vi "AlGaInPAs_prep_v00.vi"(2 "Debug Mode":bool, 3 "Elapsed Time(s)":dbl, 4 "State":enum16{"Edit", "Start", "Run", "End", "Idle"}(ring), 5 "Argument List In":string[](array[string])) -> (0 "Status Out":string, 1 "Argument List Out":string[](array[string]))   [LabVIEW 2011]
panel:
  out "AsH3?":bool
  out "PH3?":bool
  out "In?":bool
  out "Ga?":bool
  out "Al?":bool
  in  "Prep As":bool caption="Pre-run"
  out "Prep P":bool caption="Pre-run"
  in  "Prep In":bool caption="Pre-run"
  in  "Prep Ga":bool caption="Pre-run"
  in  "run_time":dbl caption="run time (s)"
  in  "prep_time":dbl caption="pre-run time (s)"
  in  "Prep Al":bool caption="Pre-run"
  in  "Run As":bool caption="Run"
  in  "AsH3 Flow":dbl caption="AsH3 Flow (0-10 sccm)" format="%.2f"
  in  "P Flow":dbl caption="P Flow (0-100 sccm)" format="%.2f"
  in  "Run P":bool caption="Run"
  in  "In Flow":dbl caption="In Flow (0-100 sscm)" format="%.2f"
  in  "Run In":bool caption="Run"
  in  "Run Ga":bool caption="Run"
  in  "Ga Flow":dbl caption="Ga Flow (0-10 sscm)" format="%.2f"
  in  "Run Al":bool caption="Run"
  in  "Al Flow":dbl caption="Al Flow (0-100 sscm)" format="%.2f"
  in  "Cancel":bool
  in  "OK":bool
  out "tTotal(s) 2":dbl
  out "tphase(s)":dbl[](array[numeric])
  out "phase":i32
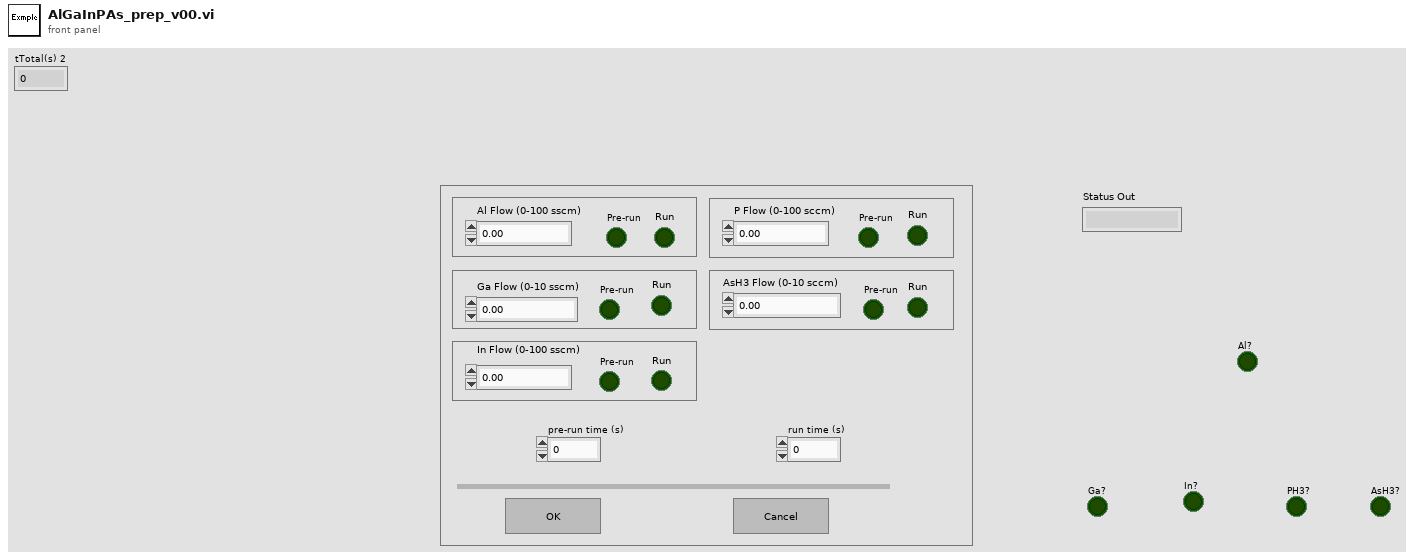
[diagram p1: front panel]
types:
  T1 = enum16{"Discrete", "Continuous", "Instantaneous"}
  T2 = enum32{"Invalid", "Default", "Floating", "Floating/Auto-Hide", "Modal"}
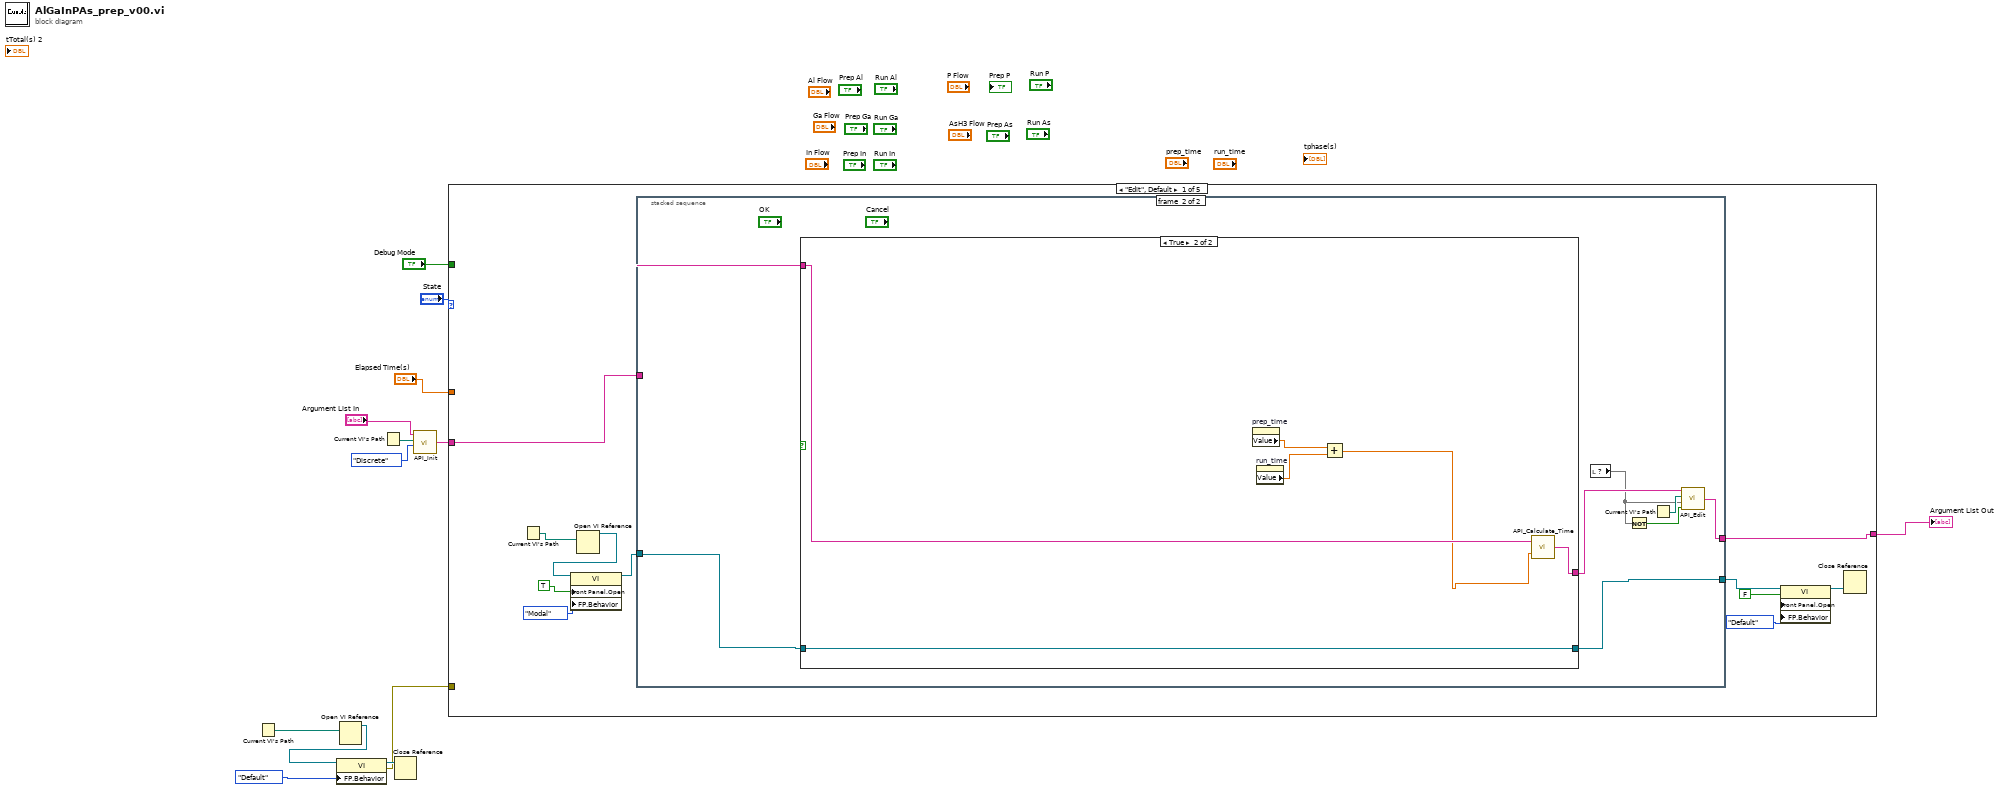
[diagram p0: block diagram]
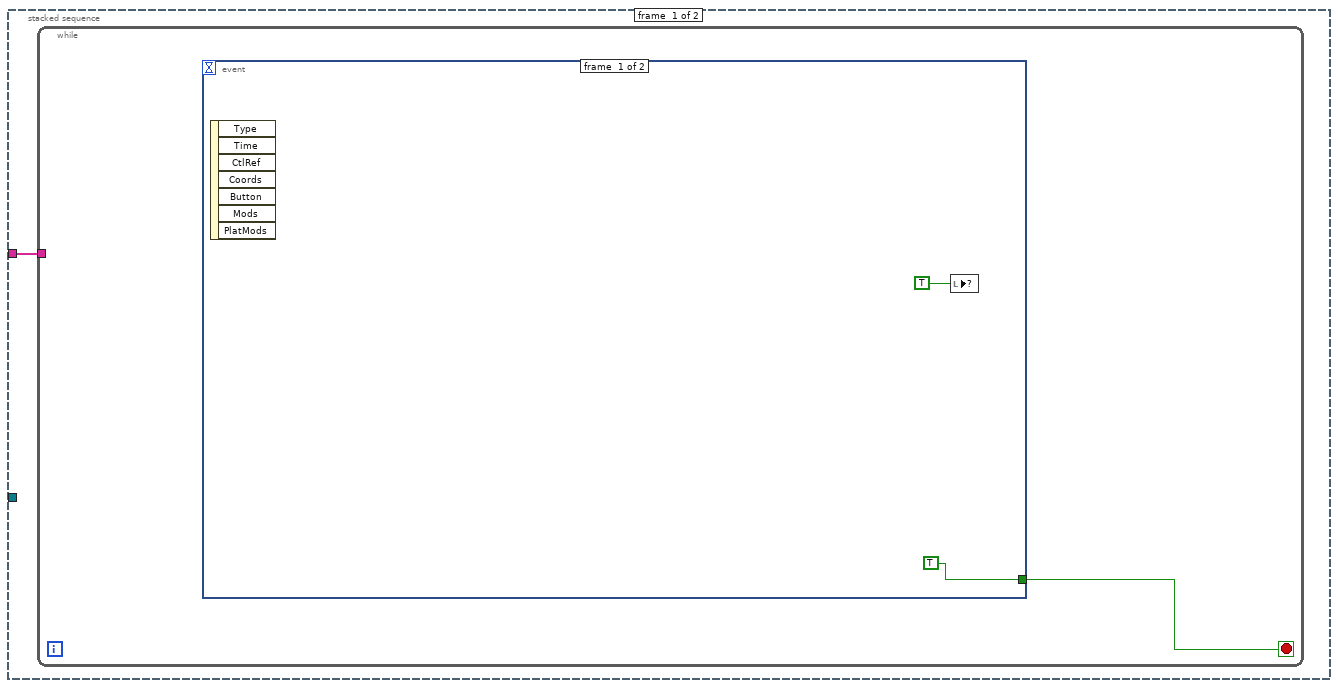
[diagram p2: hidden frame]
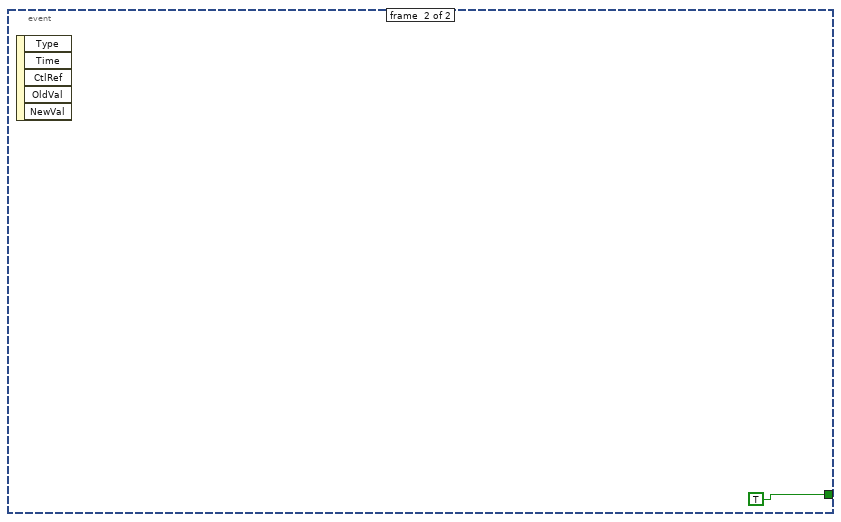
[diagram p3: hidden frame]
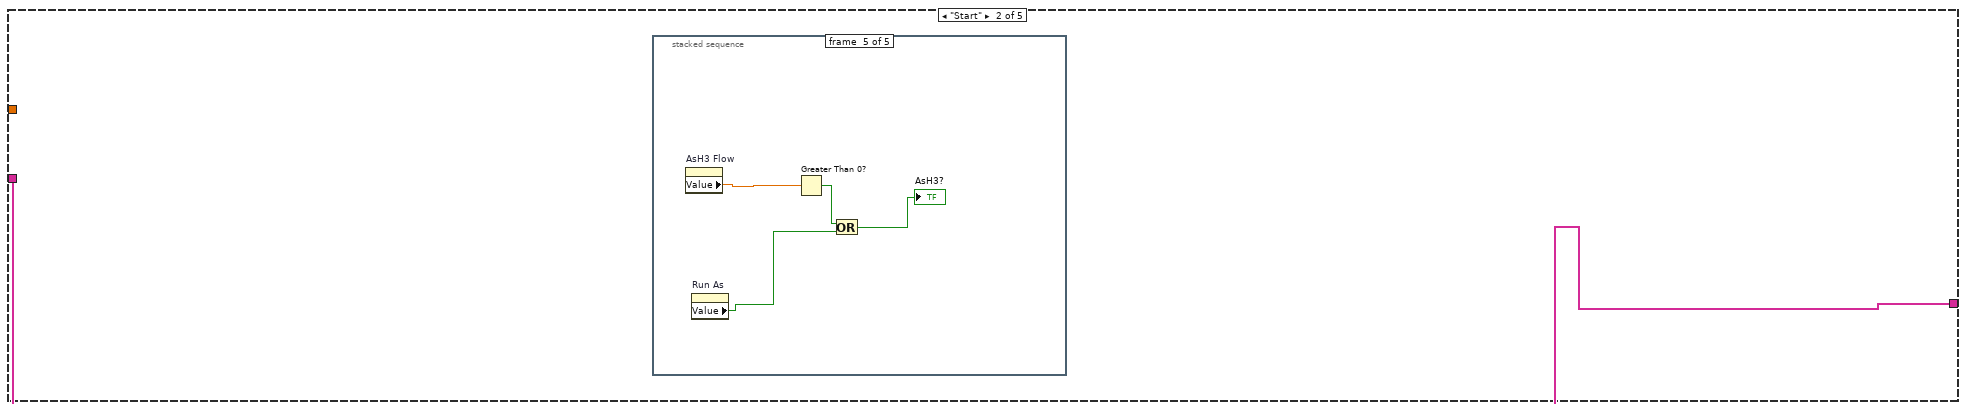
[diagram p5: hidden frame]
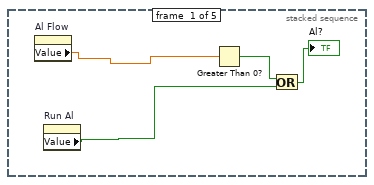
[diagram p6: hidden frame]
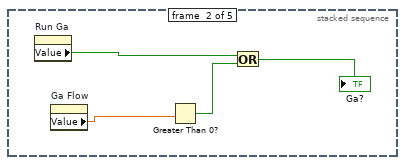
[diagram p7: hidden frame]
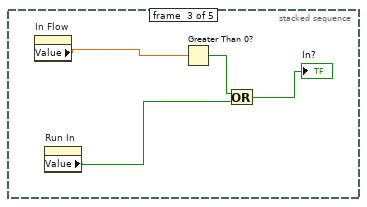
[diagram p8: hidden frame]
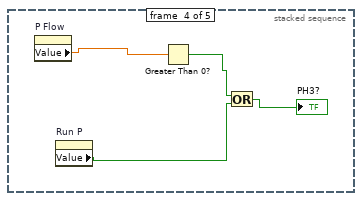
[diagram p9: hidden frame]
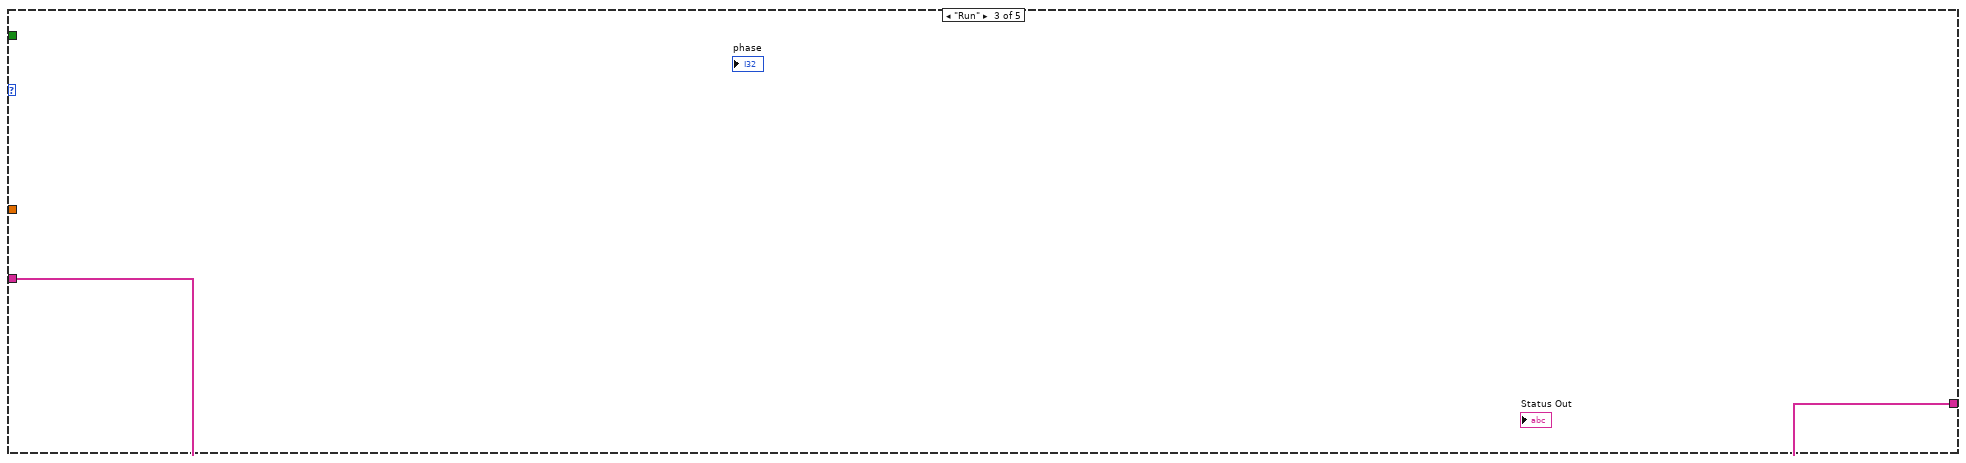
[diagram p10: hidden frame]
diagram:
  n1 = Current VI's Path() -> (path=w9:path)
  n2 = Open VI Reference(vi path=w9) -> (vi reference=w8:refnum<vi>)  [unwired: 1 in, 5 out]
  n3 = property class="VI"(reference=w8, "FP.Behavior"=T2."Default" ("Front Panel Window:Behavior")) -> (reference out=w6:refnum<vi>, error out=w5:errorcluster)  [unwired: 1 in]
  n4 = Current VI's Path() -> (path=w4:path)
  n5 = Close Reference(reference=w6) -> ()  [unwired: 1 in, 1 out]
  n6 = call "API_Init.vi"("API Mode"=T1."Discrete", "VI Path"=w4, "Argument List In"="Argument List In") -> ("Argument List Out"=w1:string[])  [unwired: 1 in]
  n7 = case shown="\"Edit\", Default" "State" {
    tunnel: "Debug Mode" -> [_ _ w70 _ _]
    tunnel: "Elapsed Time(s)" -> [_ _ w71 _ _]
    tunnel: w1 -> [w14 w47 w68 w72 w73]
    tunnel: [w21 w47 w68 w72 w73] -> w10
    tunnel: w5 -> [_ _ _ _ _]
    frame "Edit", Default {
      n8 = Current VI's Path() -> (path=w19:path)
      n9 = Open VI Reference(vi path=w19) -> (vi reference=w18:refnum<vi>)  [unwired: 1 in, 5 out]
      n10 = property class="VI"(reference=w18, "Front Panel.Open"=TRUE ("Front Panel Window:Open"), "FP.Behavior"=T2."Modal" ("Front Panel Window:Behavior")) -> (reference out=w17:refnum<vi>)  [unwired: 1 in, 1 out]
      n11 = stacked-sequence {
        tunnel: w14 -> [w25 w38]
        tunnel: w17 -> [_ w36]
        tunnel: [_ w35] -> w22
        tunnel: [_ w32] -> w21
        frame #0 {
          n12 = while {
            tunnel: w25 -> [_]
            stop <- w26 stop-if-true
            n13 = event {
              selector: _ -> [_ _]
              dyn-events: _ -> [_ _]
              timeout: _ -> [_ _]
              tunnel: [TRUE ("done_editing") TRUE ("done_editing")] -> w26
              event #0 {
                n14 = event-data() -> ()  [unwired: 1 in, 7 out]
                n15 = local write item#-1(TRUE ("is_OK")) -> ()
              }
              event #1 {
                n16 = event-data() -> ()  [unwired: 1 in, 5 out]
              }
            }
          }
        }
        frame #1 {
          n17 = case shown="True" w37 {
            tunnel: w38 -> [w40 w44]
            tunnel: [w40 w45] -> w33
            tunnel: w36 -> [w39 w46]
            tunnel: [w39 w46] -> w35
            frame False {
            }
            frame True {
              n18 = property on="prep_time" class="DigNum (strict)"() -> ("Value"=w43:dbl)  [unwired: 2 in, 2 out]
              n19 = property on="run_time" class="DigNum (strict)"() -> ("Value"=w42:dbl)  [unwired: 2 in, 2 out]
              n20 = Add(x=w43, y=w42) -> (x+y=w41:dbl)
              n21 = call "API_Calculate_Time.vi"("Time"=w41, "Argument List In"=w44) -> ("Argument List Out"=w45:string[])
            }
          }
          n22 = local read item#-1() -> (w31)
          n23 = Not(x=w31) -> (.not. x?=w30:bool)
          n24 = Current VI's Path() -> (path=w34:path)
          n25 = call "API_Edit.vi"("Cancel"=w30, "OK"=w31, "VI Path"=w34, "Argument List In"=w33) -> ("Argument List Out"=w32:string[])
        }
      }
      n26 = property class="VI"(reference=w22, "Front Panel.Open"=FALSE ("Front Panel Window:Open"), "FP.Behavior"=T2."Default" ("Front Panel Window:Behavior")) -> (reference out=w23:refnum<vi>)  [unwired: 1 in, 1 out]
      n27 = Close Reference(reference=w23) -> ()  [unwired: 1 in, 1 out]
    }
    frame "Start" {
      n28 = stacked-sequence {
        frame #0 {
          n29 = property on="Al Flow" class="DigNum (strict)"() -> ("Value"=w49:dbl)  [unwired: 2 in, 2 out]
          n30 = property on="Run Al" class="Bool (strict)"() -> ("Value"=w48:bool)  [unwired: 2 in, 2 out]
          n31 = Greater Than 0?(x=w49) -> (x > 0?=w51:bool)
          n32 = Or(x=w51, y=w48) -> (x .or. y?=→"Al?":bool)
        }
        frame #1 {
          n33 = property on="Run Ga" class="Bool (strict)"() -> ("Value"=w52:bool)  [unwired: 2 in, 2 out]
          n34 = property on="Ga Flow" class="DigNum (strict)"() -> ("Value"=w53:dbl)  [unwired: 2 in, 2 out]
          n35 = Greater Than 0?(x=w53) -> (x > 0?=w54:bool)
          n36 = Or(x=w52, y=w54) -> (x .or. y?=→"Ga?":bool)
        }
        frame #2 {
          n37 = property on="In Flow" class="DigNum (strict)"() -> ("Value"=w56:dbl)  [unwired: 2 in, 2 out]
          n38 = property on="Run In" class="Bool (strict)"() -> ("Value"=w57:bool)  [unwired: 2 in, 2 out]
          n39 = Greater Than 0?(x=w56) -> (x > 0?=w59:bool)
          n40 = Or(x=w59, y=w57) -> (x .or. y?=→"In?":bool)
        }
        frame #3 {
          n41 = property on="P Flow" class="DigNum (strict)"() -> ("Value"=w61:dbl)  [unwired: 2 in, 2 out]
          n42 = property on="Run P" class="Bool (strict)"() -> ("Value"=w60:bool)  [unwired: 2 in, 2 out]
          n43 = Greater Than 0?(x=w61) -> (x > 0?=w63:bool)
          n44 = Or(x=w63, y=w60) -> (x .or. y?=→"PH3?":bool)
        }
        frame #4 {
          n45 = property on="AsH3 Flow" class="DigNum (strict)"() -> ("Value"=w65:dbl)  [unwired: 2 in, 2 out]
          n46 = property on="Run As" class="Bool (strict)"() -> ("Value"=w64:bool)  [unwired: 2 in, 2 out]
          n47 = Greater Than 0?(x=w65) -> (x > 0?=w67:bool)
          n48 = Or(x=w67, y=w64) -> (x .or. y?=→"AsH3?":bool)
        }
      }
    }
    frame "Run" {
    }
    frame "End" {
    }
    frame "Idle" {
    }
  }
  "Argument List Out" <- w10
